vi "Initialize.vi"(0 "File Data Manager in":refnum<class "File Data Manager.lvclass">, 11 "error in (no error)":errorcluster) -> (4 "File Data Manager out":refnum<class "File Data Manager.lvclass">, 15 "error out":errorcluster)   [LabVIEW 2023, in "File Data Manager.lvlib" / "File Data Manager.lvclass"]
uses:
  File Data Manager.lvclass
  File Data Manager.lvclass/File Data Manager.ctl
  <vilib>/ActorFramework/Message Enqueuer/Init from Existing Queue.vi
  <vilib>/ActorFramework/Message Enqueuer/Message Enqueuer.lvclass
  <vilib>/ActorFramework/Actor/Actor.lvclass
  Central Data Manager/Central Data Manager Messages/Refresh Rooms Status Msg/Refresh Rooms Status Msg.lvclass
  C:/Program Files/National Instruments/LabVIEW 2023/vi.lib/ActorFramework/Actor/Actor.lvclass
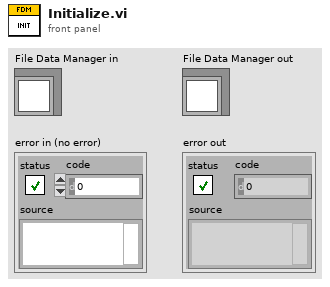
[diagram p1: front panel]
types:
  T1 = typedef "Central Data Manager.lvlib/Central Data Manager.lvclass/Room Size Details.ctl" = cluster{"Size":string, "Cost Per Day (Rs)":u32, "Occupancy Limit (Adult)":u32, "Occupancy Limit (Children)":u32}
  T2 = typedef "Central Data Manager.lvlib/Central Data Manager.lvclass/Room Details.ctl" = cluster{"Room No":string, "Room Size":string, "Room Occupancy Status":T3, "Guest Details":T4, "Occupancy Count (Adult)":u32, "Occupancy Count (Children)":u32, "Check-in Time":timestamp, "Check-out Time":timestamp}
  T3 = typedef "Central Data Manager.lvlib/Central Data Manager.lvclass/Room Occupancy Status.ctl" = enum16{"Not Occupied", "Occupied", "Under Maintainance", "Not Servicable"}
  T4 = typedef "Central Data Manager.lvlib/Central Data Manager.lvclass/Guest Details.ctl" = cluster{"Contact Number":string, "Primary Guest Name":string}
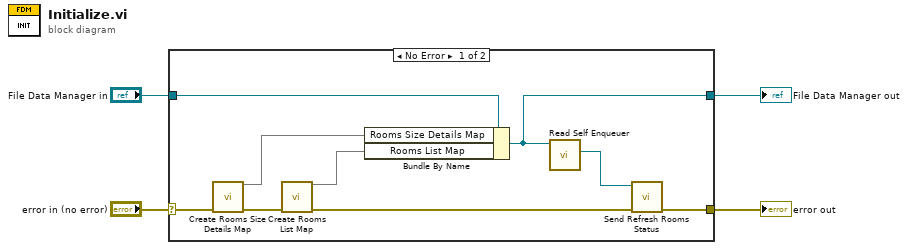
[diagram p0: block diagram]
diagram:
  n1 = case shown="No Error" "error in (no error)" {
    selector: "error in (no error)" -> [w12 w14]
    tunnel: "File Data Manager in" -> [w13 w15]
    tunnel: [w8 w15] -> w3
    tunnel: [w6 w14] -> w1
    frame No Error {
      n2 = call "Create Rooms Size Details Map.vi"("error in (no error)"=w12) -> ("Rooms Size Details Map"=w10:map{string, T1}, "error out"=w11:errorcluster)  [unwired: 13 in]
      n3 = call "Create Rooms List Map.vi"("error in (no error)"=w11) -> ("Rooms List Map"=w9:map{string, T2}, "error out"=w7:errorcluster)  [unwired: 13 in]
      n4 = Bundle By Name(cluster=w13, "Rooms Size Details Map"=w10, "Rooms List Map"=w9) -> (w8:refnum<class "File Data Manager.lvclass">)
      n5 = call <vilib>:"Read Self Enqueuer.vi"("Actor"=w8) -> ("Self Enqueuer"=w5:refnum<class "Message Enqueuer.lvclass">)  [unwired: 10 in]
      n6 = call "Send Refresh Rooms Status.vi"("error in (no error)"=w7, "Message Enqueuer"=w5) -> ("error out"=w6:errorcluster)  [unwired: 8 in, 1 out]
    }
    frame Error {
    }
  }
  "error out" <- w1
  "File Data Manager out" <- w3
